vi "Clear.vi"(8 "error in (no error)":errorcluster, 11 "Mock Instrument Interface In":refnum<class "Mock Instrument Interface.lvclass">) -> (0 "error out":errorcluster, 3 "Mock Instrument Interface Out":refnum<class "Mock Instrument Interface.lvclass">)   [LabVIEW 2020, in "Low Level PSU With Tests.lvlib" / "Mock Instrument Interface.lvclass"]
uses:
  Mock Instrument Interface.lvclass
  Mock Instrument Interface.lvclass/Mock Instrument Interface.ctl
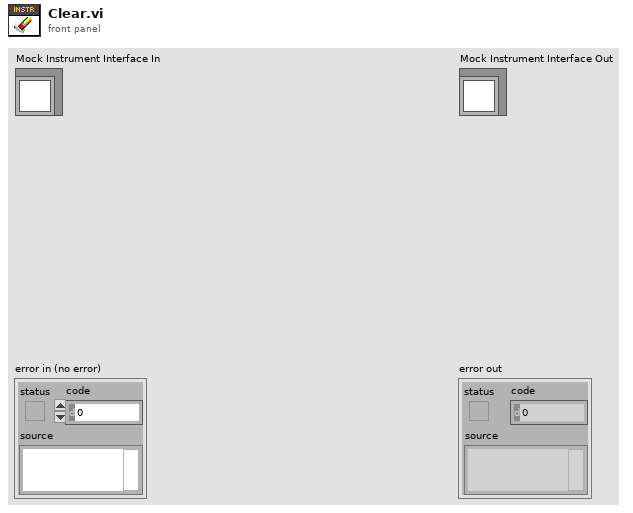
[diagram p1: front panel]
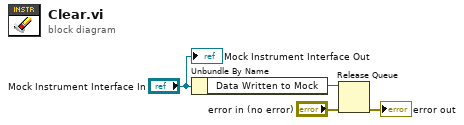
[diagram p0: block diagram]
diagram:
  n1 = Unbundle By Name("Mock Instrument Interface In") -> ("Data Written to Mock"=w1:refnum<queue>)
  n2 = Release Queue(queue=w1, error in (no error)="error in (no error)") -> (error out=→"error out":errorcluster)  [unwired: 1 in, 2 out]
  "Mock Instrument Interface Out" <- "Mock Instrument Interface In"
